vi "Wait on chirps generation.vi"(8 "error in (no error)":errorcluster, 11 "Imaging Protocol":T1) -> (0 "error out":errorcluster, 3 "Timed out waiting on Chirps generation":bool)   [LabVIEW 2020]
uses:
  Typedefs/Imaging Protocols enum.ctl
  Typedefs/Set Main VI cursor.ctl
  Global Variables/gl_UI Ctrl Refs.vi
  Global Variables/General Globals.vi
panel:
  out "Elapsed Time (s)":dbl
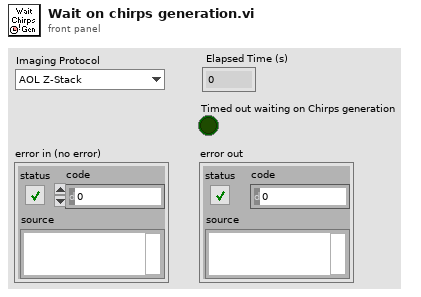
[diagram p1: front panel]
types:
  T1 = typedef "Imaging Protocols enum.ctl" = enum16{"AOL Z-Stack", "Motor Z Stack", "Functional Acquisition", "Single Plane Acquisition", "Volume Acquisition", "Live Imaging", "Live Plane Imaging", "Live Volume Imaging"}
  T2 = typedef "Set Main VI cursor.ctl" = enum16{"Release busy cursor", "Set busy cursor"}
  T3 = typedef "UI ctrl refs cluster.ctl" = cluster{"Top level VI path":path, "Top level VI ref":refnum<vi>, "User menu ref":refnum<k9>, "Sub Panel control":refnum<vi>, "Imaging Param Tab":refnum<vi>, "Occurrence-Start drivers":refnum<k4>, "Occurrence-Speed logging initialised":refnum<k4>, "Occurrence-XYZ stage initialised":refnum<k4>, "Exit button":refnum<vi>, "Status ind":refnum<vi>, "Set as origin":refnum<vi>, "Speed Logging":refnum<vi>, "Time Lapse":refnum<vi>, "Live Imaging":refnum<vi>, "AOL Z Stack":refnum<vi>, "Motor Z Stack":refnum<vi>, "Funct Acq button":refnum<vi>, "Hard Shutter":refnum<vi>, "Virtual Shutter":refnum<vi>, "Laser Power":refnum<vi>, "AOL Mode":refnum<vi>, "Frame Size":refnum<vi>, "Field of View":refnum<vi>, "Dwell Time":refnum<vi>, "Zoom":refnum<vi>, "AOL Z":refnum<vi>, "Objective":refnum<vi>, "Axis":refnum<vi>, "Paths & Names":refnum<vi>, "Experiment folder path (ind.)":refnum<vi>, "Last State (Ind.)":refnum<vi>, "Averages":refnum<vi>, "Angle (degrees)":refnum<vi>, "X centre":refnum<vi>, "Y centre":refnum<vi>, "Plane Mode":refnum<vi>, "# Planes":refnum<vi>, "Z Start":refnum<vi>, "Z Stop":refnum<vi>, "Z Step":refnum<vi>, "PMT 1":refnum<vi>, "PMT 2":refnum<vi>, "Stage XYZ Position":refnum<vi>, "Pockels@Z Start":refnum<vi>, "Pockels@Z Stop":refnum<vi>, "Obtain Z Start":refnum<vi>, "Obtain Z Stop":refnum<vi>, "Live stim.trig.period":refnum<vi>, "Live stim.trig.enable":refnum<vi>, "Movement Correction":refnum<vi>, "Load Reference Image":refnum<vi>, "XY Stage Move":refnum<vi>, "MovCor Cluster":refnum<vi>, "RefDAQParam":refnum<vi>, "Funct. Acq. Pockels Modulation":refnum<vi>, "Ref Laser Power":refnum<vi>, "Enable Video Recording":refnum<vi>, "Video Record-Live Imaging":refnum<vi>, "Video Record-Funct acq":refnum<vi>, "Reference Source":refnum<vi>, "AOL Z-stack Chirps Ready (ind)":refnum<vi>, "Target time between mov.cor. ref triggers (ms)":refnum<vi>, "Funct. Acq. Ref frame save":refnum<vi>, "Tracking button":refnum<vi>, "Show ref plots window":refnum<vi>, "Center freq ind (nm)":refnum<vi>, "Pickup mode (ind)":refnum<vi>, "Logging queue (ind)":refnum<vi>, "Back aperture power (ind.)":refnum<vi>, "Power after objective (ind.)":refnum<vi>, "Switch user":refnum<vi>, "Ls1 Conn. Status":refnum<vi>, "Ls1Tuning Status":refnum<vi>, "Ls1 Faults":refnum<vi>, "Ls1 Connection":refnum<vi>, "Ls1 Mode":refnum<vi>, "Ls1 POWER [mW]":refnum<vi>, "Ls1Shutter":refnum<vi>, "Ls1 Wavelength":refnum<vi>, "Ls1 Note":refnum<vi>, "Ls1 Confirm Wav":refnum<vi>, "Ls1 PreChrp Prism1":refnum<vi>, "Ls1 PreChrp Prism2":refnum<vi>, "Ls1 wav top Ind":refnum<vi>, "Ls1 power top Ind":refnum<vi>, "Ls1 Pump peak Hold":refnum<vi>, "Ls1 Status Ind":refnum<vi>, "Ls1 wav cancel":refnum<vi>, "Experiment Type":refnum<vi>, "Biology Information":refnum<vi>, "Camera recording status":refnum<vi>}
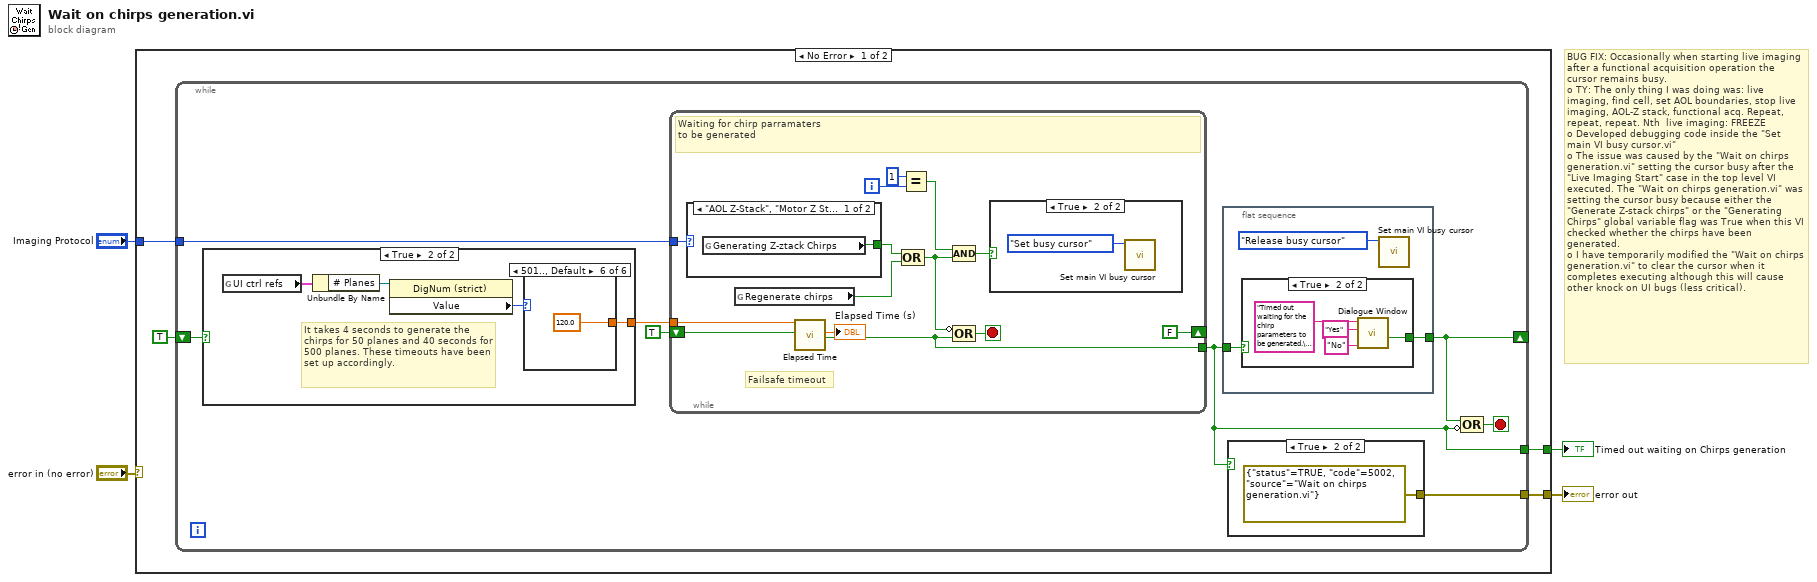
[diagram p0: block diagram]
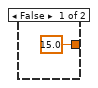
[diagram p3: hidden frame]
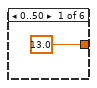
[diagram p4: hidden frame]
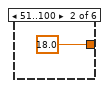
[diagram p5: hidden frame]
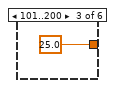
[diagram p6: hidden frame]
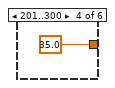
[diagram p7: hidden frame]
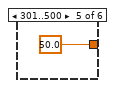
[diagram p8: hidden frame]
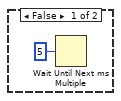
[diagram p10: hidden frame]
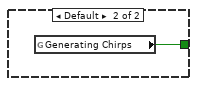
[diagram p11: hidden frame]
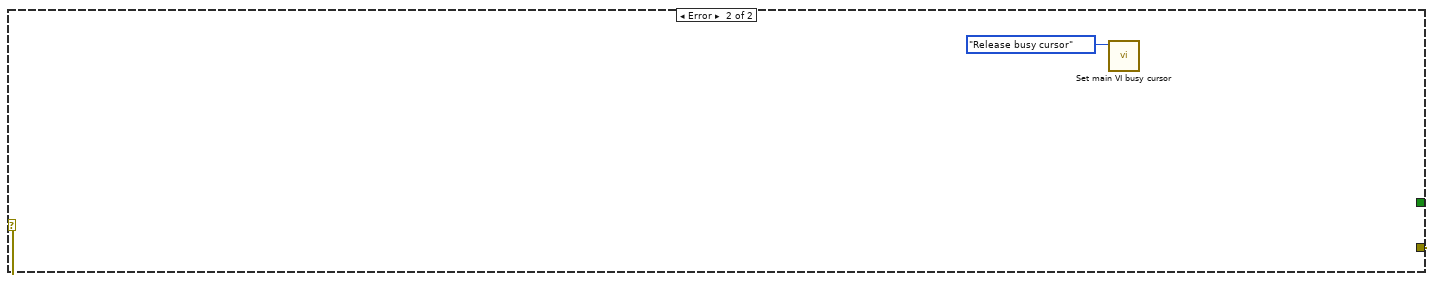
[diagram p12: hidden frame]
diagram:
  # "BUG FIX: Occasionally when starting live imaging after a functional acquisition operation the cursor remains busy.\no\tTY: The only thing I was doing was: live imaging, find cell, set AOL boundaries, stop live imaging, AOL-Z stack, functional acq. Repeat, repeat, repeat. Nth  live imaging: FREEZE\no\tDeveloped debugging code inside the \"Set main VI busy cursor.vi\"\no\tThe issue was caused by the \"Wait on chirps generation.vi\" setting the cursor busy after the \"Live Imaging Start\" case in the top level VI executed. The \"Wait on chirps generation.vi\" was setting the cursor busy because either the \"Generate Z-stack chirps\" or the \"Generating Chirps\" global variable flag was True when this VI checked whether the chirps have been generated.\no\tI have temporarily modified the \"Wait on chirps generation.vi\" to clear the cursor when it completes executing although this will cause other knock on UI bugs (less critical)."
  n1 = case shown="No Error" "error in (no error)" {
    selector: "error in (no error)" -> [_ w55]
    tunnel: [w5 w55] -> w2
    tunnel: [w7 _] -> w1
    tunnel: "Imaging Protocol" -> [w8 _]
    frame No Error {
      n2 = while {
        tunnel: w8 -> [w16]
        tunnel: [w10] -> w7
        shift-right: [w9] -> _
        shift-left: TRUE -> [w12]
        tunnel: [w11] -> w5
        stop <- w13 stop-if-true
        n3 = case shown="True" w12 {
          tunnel: [15.0 ("Time Target (s)") w19] -> w14
          frame False {
          }
          frame True {
            # "It takes 4 seconds to generate the chirps for 50 planes and 40 seconds for 500 planes. These timeouts have been set up accordingly."
            n4 = global read "gl_UI Ctrl Refs.vi" "UI ctrl refs"() -> (w22:T3)
            n5 = Unbundle By Name(w22) -> ("# Planes"=w21:refnum<vi>)
            n6 = property class="DigNum (strict)"(reference=w21) -> ("Value"=w20:u16)  [unwired: 1 in, 2 out]
            n7 = case shown="501.., Default" w20 {
              tunnel: [13.0 ("Time Target (s)") 18.0 ("Time Target (s)") 25.0 ("Time Target (s)") 35.0 ("Time Target (s)") 50.0 ("Time Target (s)") 120.0 ("Time Target (s)")] -> w19
              frame 0..50 {
              }
              frame 51..100 {
              }
              frame 101..200 {
              }
              frame 201..300 {
              }
              frame 301..500 {
              }
              frame 501.., Default {
              }
            }
          }
        }
        n8 = while {
          shift-right: [FALSE] -> _
          shift-left: TRUE -> [w49]
          tunnel: [w46] -> w10
          tunnel: w16 -> [w45]
          tunnel: w14 -> [w36]
          i -> [w44]
          stop <- w47 stop-if-true
          # "Failsafe timeout"
          # "Waiting for chirp parramaters\nto be generated"
          n9 = case shown="\"AOL Z-Stack\", \"Motor Z Stack\"" w45 {
            tunnel: [w52 w53] -> w40
            frame "AOL Z-Stack", "Motor Z Stack" {
              n10 = global read "General Globals.vi" "Generating Z-ztack Chirps"() -> (w52:bool)
            }
            frame Default {
              n11 = global read "General Globals.vi" "Generating Chirps"() -> (w53:bool)
            }
          }
          n12 = global read "General Globals.vi" "Regenerate chirps"() -> (w39:bool)
          n13 = call "Elapsed Time"("Time Target (s)"=w36, "Reset"=w49) -> ("Elapsed Time (s)"=→"Elapsed Time (s)":dbl, "Time has Elapsed"=w46:bool)  [unwired: 10 in, 6 out]
          n14 = Equal?(x=1, y=w44) -> (x = y?=w42:bool)
          n15 = Compound Arithmetic op=OR(w40, w39) -> (w38:bool)
          n16 = Compound Arithmetic op=AND(w42, w38) -> (w41:bool)
          n17 = Compound Arithmetic op=OR(invert w38, w46) -> (w47:bool)
          n18 = case shown="True" w41 {
            frame False {
              n19 = Wait Until Next ms Multiple(millisecond multiple=u32 5) -> ()  [unwired: 1 out]
            }
            frame True {
              n20 = call "Set main VI busy cursor.vi"("Main VI's cursor"=Set_Main_VI_cursor."Set busy cursor") -> ()  [unwired: 10 in, 1 out]
            }
          }
        }
        n21 = flat-sequence {
          tunnel: w10 -> [w31]
          tunnel: [w30] -> w9
          frame #0 {
            n22 = case shown="True" w31 {
              tunnel: [_ w32] -> w30
              frame False {
              }
              frame True {
                n23 = call "Dialogue Window.vi"("Caption-Left button (Cancel)"="No", "Caption-Right button (OK)"="Yes", "Message string"="Timed out waiting for the chirp parameters to be generated.\n\nWait a little longer?") -> ("Cancelled (Left button pressed)"=w32:bool)  [unwired: 6 in, 2 out]
              }
            }
            n24 = call "Set main VI busy cursor.vi"("Main VI's cursor"=Set_Main_VI_cursor."Release busy cursor") -> ()  [unwired: 10 in, 1 out]
          }
        }
        n25 = case shown="True" w10 {
          tunnel: [_ errorcluster {"status"=TRUE, "code"=5002, "source"="Wait on chirps generation.vi"} ("error IO")] -> w11
          frame False {
          }
          frame True {
          }
        }
        n26 = Compound Arithmetic op=OR(w9, invert w10) -> (w13:bool)
      }
    }
    frame Error {
      n27 = call "Set main VI busy cursor.vi"("Main VI's cursor"=Set_Main_VI_cursor."Release busy cursor") -> ()  [unwired: 10 in, 1 out]
    }
  }
  "error out" <- w2
  "Timed out waiting on Chirps generation" <- w1
